vi "Autonomous Independent.vi"() -> ()   [LabVIEW 2016]
doc: "This VI is called when autonomous begins, and will automatically be terminated when autonomous ends. You can carry out timed or sensor driven robot movement independently without needing to return to the caller."
uses:
  <vilib>/Rock Robotics/Network Tables/NT Read String.vi
  Robot Global Data.vi
  <vilib>/Rock Robotics/Network Tables/NT Read Number.vi
  <vilib>/Rock Robotics/Network Tables/NT Write Number.vi
  <vilib>/Rock Robotics/Network Tables/NT Read Boolean.vi
  <vilib>/Rock Robotics/WPI/Utilities/WPI_GetSetVariantRefNum.vi
  <vilib>/Rock Robotics/WPI/ThirdParty/Sensors/ADIS16448 IMU/ADIS16448_IMU.lvlib
panel:
  out "Numeric":i32
  out "Reset":bool
  # "Be sure to right-click and choose Data Operations>>Make Current Value default if you want to save the array values with the VI"
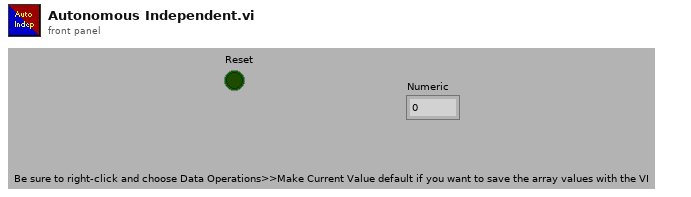
[diagram p1: front panel]
types:
  T1 = typedef "WPI_EncoderDevRef.ctl" = cluster{"DevStatus":errorcluster, "EncoderIndex":T2, "CounterIndex":T3, "DistancePerCount":dbl, "Decoding Type":T4}
  T2 = typedef "FPGA_EncoderIdx.ctl" = enum8{"Enc 0", "Enc 1", "Enc 2", "Enc 3", "Enc 4", "Enc 5", "Enc 6", "Enc 7", "Invalid"}
  T3 = typedef "FPGA_CounterCtrSystemIndex.ctl" = enum8{"Ctr 0", "Ctr 1", "Ctr 2", "Ctr 3", "Ctr 4", "Ctr 5", "Ctr 6", "Ctr 7", "Invalid"}
  T4 = typedef "WPI_EncoderType.ctl" = enum16{"1x", "2x", "4x"}
  T5 = typedef "WPI_GyroDevRef.ctl" = cluster{"DevStatus":errorcluster, "Analog Channel":T6, "Offset":dbl, "Gain (VoltsPerDegree/Second)":dbl, "Gyro Type":enum16{"Analog", "XRS450"}, "Handle":i32, "SPI Bus":T7, "Device Found":bool, "Sample Rate":dbl, "Calibrate On Open":bool}
  T6 = typedef "FPGA_AIChannel.ctl" = enum8{"AI 0", "AI 1", "AI 2", "AI 3", "AI MXP 0", "AI MXP 1", "AI MXP 2", "AI MXP 3", "Invalid"}
  T7 = typedef "spi_bus.ctl" = enum16{"SPI On-Board, CS0", "SPI On-Board, CS1", "SPI On-Board, CS2", "SPI On-Board, CS3", "SPI MXP", "Invalid"}
  T8 = typedef "ADIS16448_IMU.lvlib/ADI_IMU_ADIS16448_InterruptDevRef.ctl" = cluster{"ADI IMU DevRef":T9, "InterruptRef":T10}
  T9 = typedef "ADIS16448_IMU.lvlib/ADI_IMU_ADIS16448_IMUDevRef.ctl" = cluster{"DevStatus":errorcluster, "Handle":i32, "SPI Bus":T7, "Device Found":bool, "Device Ready":bool, "Yaw Axis":enum16{"X", "Y", "Z"}, "AHRS Algorithm":enum16{"Complementary", "Madgwick"}, "Serial":u16, "Lot ID 2":u16, "Lot ID 1":u16, "Product ID":u16}
  T10 = typedef "WPI_InterruptRef.ctl" = cluster{"DevStatus":errorcluster, "InterruptIndex":T11}
  T11 = typedef "FPGA_InterruptIndex.ctl" = enum8{"0", "1", "2", "3", "4", "5", "6", "7", "Invalid"}
  T12 = typedef "WPI_RobotDriveDevRef.ctl" = cluster{"DevStatus":errorcluster, "Motors[]":T13[], "Square Inputs":bool, "Max Output":dbl}
  T13 = typedef "WPI_MotorControlDeviceRef.ctl" = cluster{"DeviceStatus":errorcluster, "Type":T14, "PWM":cluster{"PWM Channel":T15, "DeadBand":T16}, "CAN":cluster{"Device Number":u8, "SetOutput VI Ref":variant, "GetOutput VI Ref":variant, "Enable VI Ref":variant, "Disable VI Ref":variant, "Data":variant}, "Invert":bool}
  T14 = typedef "WPI_MotorControlType.ctl" = enum16{"PWM", "CAN"}
  T15 = typedef "FPGA_DIOPWMChannel.ctl" = enum8{"PWM 0", "PWM 1", "PWM 2", "PWM 3", "PWM 4", "PWM 5", "PWM 6", "PWM 7", "PWM 8", "PWM 9", "PWM MXP 0", "PWM MXP 1", "PWM MXP 2", "PWM MXP 3", "PWM MXP 4", "PWM MXP 5", "PWM MXP 6", "PWM MXP 7", "PWM MXP 8", "PWM MXP 9", "Invalid"}
  T16 = typedef "WPI_PWMDeadband.ctl" = cluster{"Name":string, "maxPositivePwm":i32, "minPositivePwm":i32, "centerPwm":i32, "maxNegativePwm":i32, "minNegativePwm":i32, "angularRange":u16}
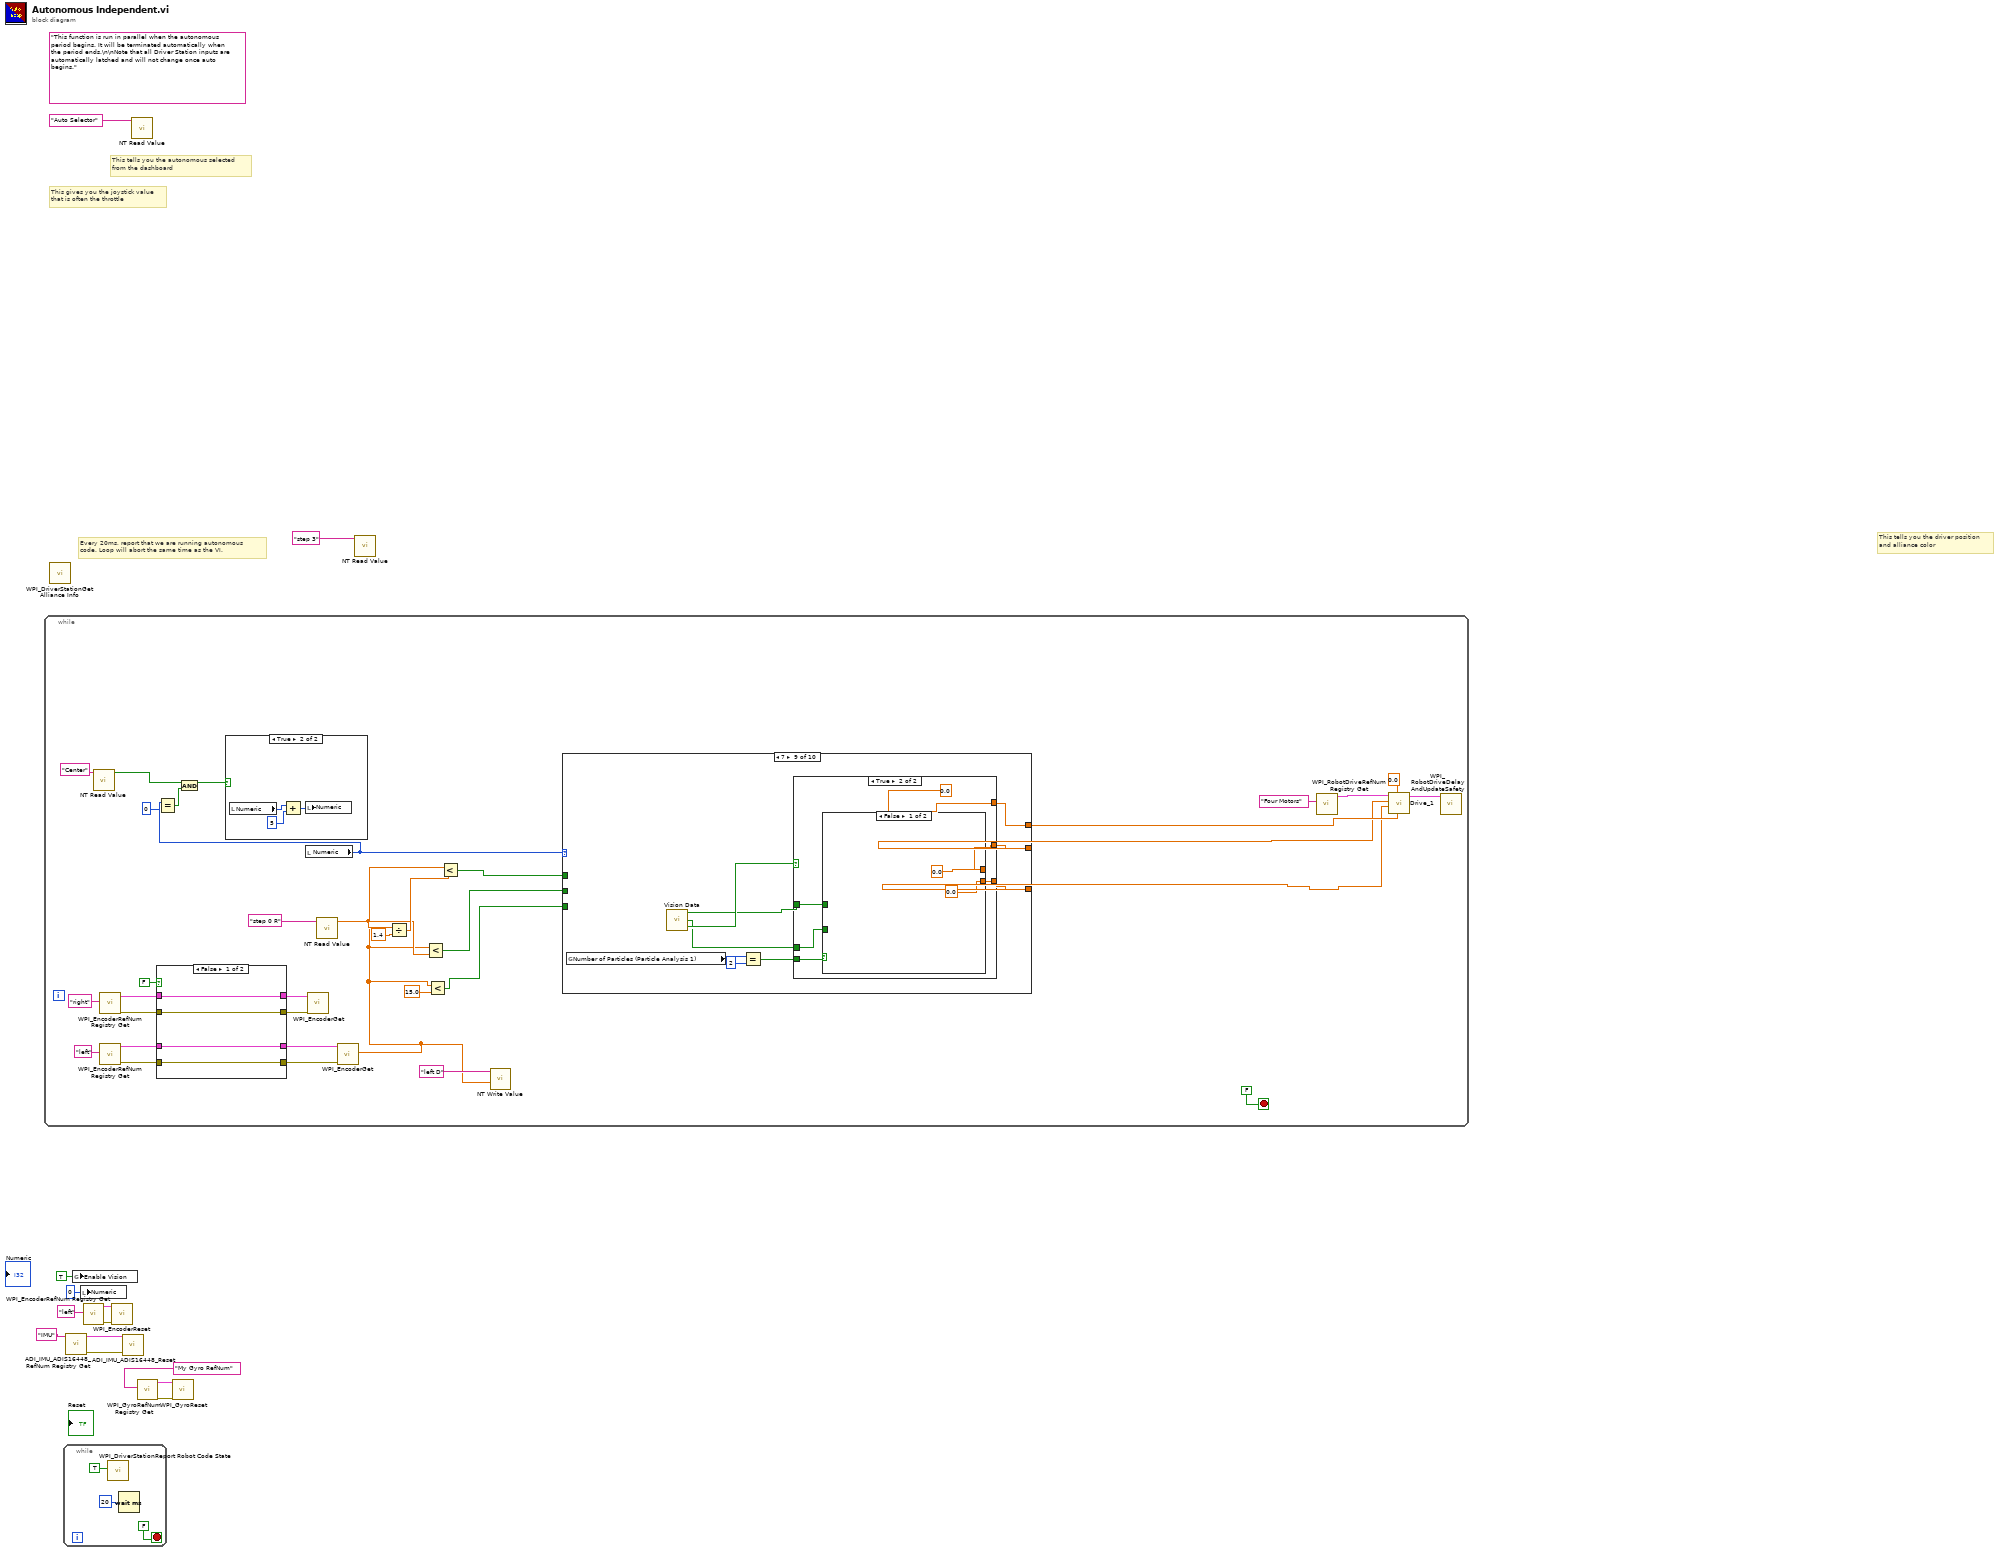
[diagram p0: block diagram]
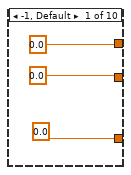
[diagram p3: hidden frame]
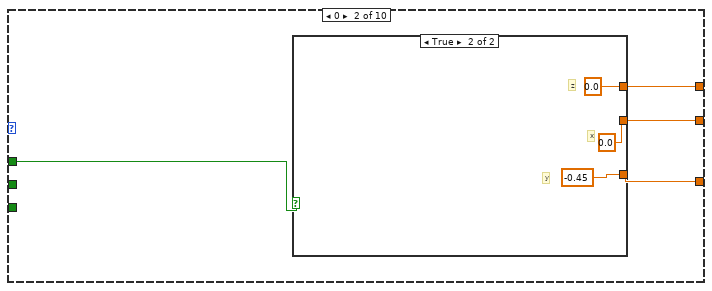
[diagram p4: hidden frame]
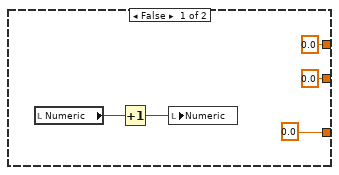
[diagram p5: hidden frame]
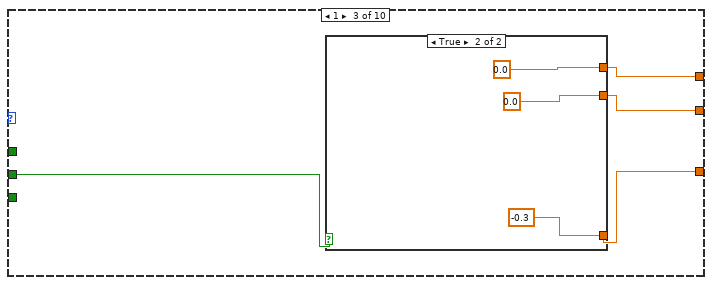
[diagram p6: hidden frame]
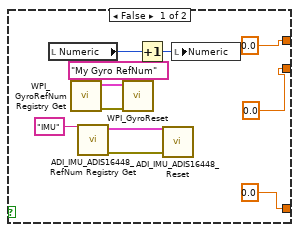
[diagram p7: hidden frame]
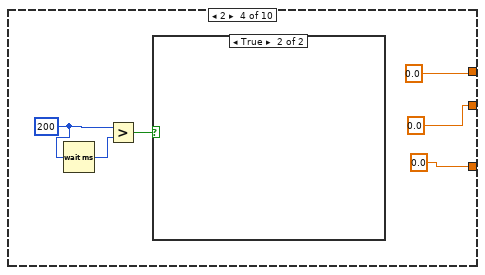
[diagram p8: hidden frame]
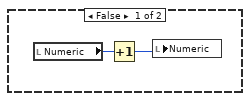
[diagram p9: hidden frame]
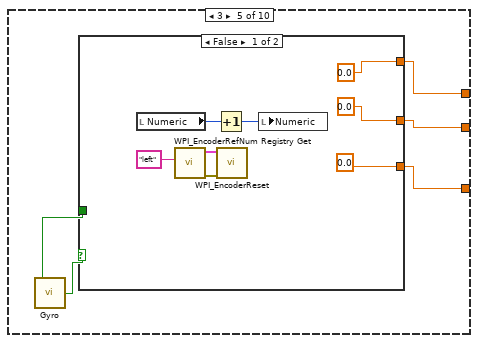
[diagram p10: hidden frame]
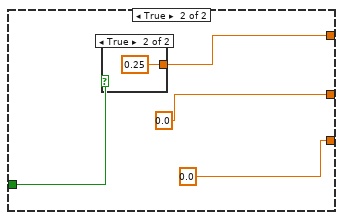
[diagram p11: hidden frame]
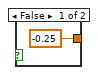
[diagram p12: hidden frame]
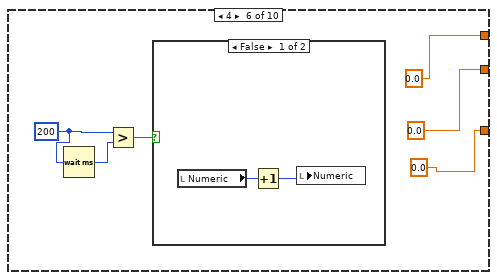
[diagram p13: hidden frame]
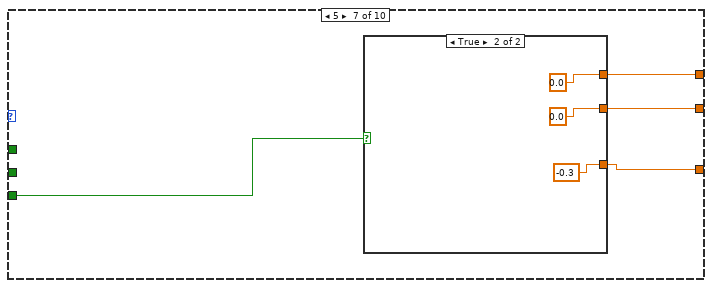
[diagram p15: hidden frame]
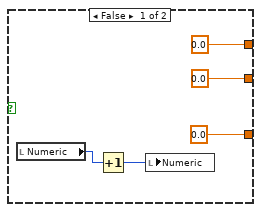
[diagram p16: hidden frame]
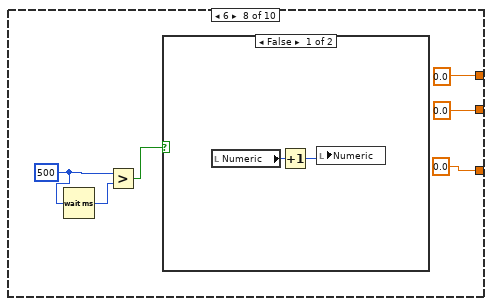
[diagram p17: hidden frame]
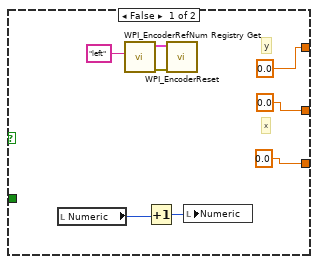
[diagram p19: hidden frame]
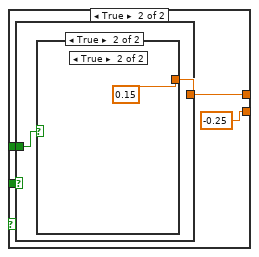
[diagram p20: hidden frame]
diagram:
  (unwired) "This function is run in parallel when the autonomous period begins. It will be terminated automatically when the period ends.\n\nNote that all Driver Station inputs are automatically latched and will not change once auto begins."
  # "This tells you the autonomous selected\nfrom the dashboard"
  # "Every 20ms, report that we are running autonomous\ncode. Loop will abort the same time as the VI."
  # "This gives you the joystick value\nthat is often the throttle"
  # "This tells you the driver position\nand alliance color"
  n1 = while {
    stop <- FALSE stop-if-true
    n2 = call-poly <vilib>:"NT Read Value.vi"("Name"="Center") -> ("Boolean"=w18:bool)  [unwired: 9 in, 1 out]
    n3 = call <vilib>:"WPI_EncoderRefNum Registry Get.vi"("refnum name"="right") -> ("error out"=w40:errorcluster, "EncoderDevRef"=w42:T1)  [unwired: 9 in]
    n4 = call <vilib>:"WPI_EncoderRefNum Registry Get.vi"("refnum name"="left") -> ("error out"=w46:errorcluster, "EncoderDevRef"=w47:T1)  [unwired: 9 in]
    n5 = case shown="False" FALSE {
      tunnel: w47 -> [w180 w188]
      tunnel: w46 -> [w179 w187]
      tunnel: [w180 w186] -> w45
      tunnel: [w179 w185] -> w44
      tunnel: [w178 w183] -> w43
      tunnel: w42 -> [w178 w184]
      tunnel: [w177 w182] -> w41
      tunnel: w40 -> [w177 w181]
      frame False {
      }
      frame True {
        n6 = call <vilib>:"WPI_EncoderReset.vi"("error in (no error)"=w181, "EncoderDevRef"=w184) -> ("error out"=w182:errorcluster, "EncoderDevRef"=w183:T1)  [unwired: 8 in]
        n7 = call <vilib>:"WPI_EncoderReset.vi"("error in (no error)"=w187, "EncoderDevRef"=w188) -> ("error out"=w185:errorcluster, "EncoderDevRef"=w186:T1)  [unwired: 8 in]
      }
    }
    n8 = local read "Numeric"() -> (w15:i32)
    n9 = Equal?(x=w15, y=0) -> (x = y?=w16:bool)
    n10 = And(x=w18, y=w16) -> (x .and. y?=w17:bool)
    n11 = case shown="True" w17 {
      frame False {
      }
      frame True {
        n12 = local read "Numeric"() -> (w51:i32)
        n13 = Add(x=w51, y=5 ("x")) -> (x+y=w49:i32)
        n14 = local write "Numeric"(w49) -> ()
      }
    }
    n15 = call <vilib>:"WPI_EncoderGet.vi"("error in (no error)"=w41, "EncoderDevRef"=w43) -> ()  [unwired: 4 in, 6 out]
    n16 = call-poly <vilib>:"NT Read Value.vi"("Name"="step 0 R") -> ("Numeric"=w32:dbl)  [unwired: 9 in, 1 out]
    n17 = call <vilib>:"WPI_EncoderGet.vi"("error in (no error)"=w44, "EncoderDevRef"=w45) -> ("Distance"=w22:dbl)  [unwired: 4 in, 5 out]
    n18 = Divide(x=w32, y=1.4) -> (x/y=w34:dbl)
    n19 = Less?(x=w22, y=w32) -> (x < y?=w24:bool)
    n20 = Less?(x=w22, y=15.0) -> (x < y?=w20:bool)
    n21 = Less?(x=w22, y=w34) -> (x < y?=w28:bool)
    n22 = call-poly <vilib>:"NT Write Value.vi"("Numeric"=w22, "Name"="left D") -> ()  [unwired: 9 in, 1 out]
    n23 = case shown="7" w15 {
      tunnel: [0.0 w58 w70 0.0 w97 0.0 w122 0.0 w146 0.0] -> w27
      tunnel: [0.0 w57 w69 0.0 w96 0.0 w121 0.0 w145 0.0] -> w26
      tunnel: [0.0 w56 w68 0.0 w95 0.0 w120 0.0 w144 -0.2] -> w25
      tunnel: w28 -> [_ w55 _ _ _ _ _ _ _ _]
      tunnel: w24 -> [_ _ w67 _ _ _ _ _ _ _]
      tunnel: w20 -> [_ _ _ _ _ _ w123 _ _ _]
      frame -1, Default {
      }
      frame 0 {
        n24 = case shown="True" w55 {
          tunnel: [0.0 0.0] -> w57
          tunnel: [0.0 0.0] -> w58
          tunnel: [0.0 -0.45] -> w56
          frame False {
            n25 = local read "Numeric"() -> (w59:i32)
            n26 = Increment(x=w59) -> (x+1=w60:i32)
            n27 = local write "Numeric"(w60) -> ()
          }
          frame True {
            # "y"
            # "x"
            # "z"
          }
        }
      }
      frame 1 {
        n28 = case shown="True" w67 {
          tunnel: [0.0 -0.3] -> w68
          tunnel: [0.0 0.0] -> w70
          tunnel: [0.0 0.0] -> w69
          frame False {
            n29 = local read "Numeric"() -> (w74:i32)
            n30 = call <vilib>:"WPI_GyroRefNum Registry Get.vi"("refnum name"="My Gyro RefNum") -> ("error out"=w76:errorcluster, "GyroDevRef"=w77:T5)  [unwired: 9 in]
            n31 = call <vilib>:"ADI_IMU_ADIS16448_RefNum Registry Get.vi"("refnum name"="IMU") -> ("error out"=w80:errorcluster, "ADI IMU Interrupt DevRef"=w79:T8)  [unwired: 9 in]
            n32 = call <vilib>:"WPI_GyroReset.vi"("error in"=w76, "GyroDevRef"=w77) -> ()  [unwired: 8 in, 2 out]
            n33 = Increment(x=w74) -> (x+1=w75:i32)
            n34 = call <vilib>:"ADI_IMU_ADIS16448_Reset.vi"("error in"=w80, "ADI IMU Interrupt DevRef"=w79) -> ()  [unwired: 8 in, 2 out]
            n35 = local write "Numeric"(w75) -> ()
          }
          frame True {
          }
        }
      }
      frame 2 {
        w86 = u32 200 ("x")
        n36 = Wait (ms)(milliseconds to wait=w86) -> (millisecond timer value=w87:u32)
        n37 = Greater?(x=w86, y=w87) -> (0:w85:bool)
        n38 = case shown="True" w85 {
          frame False {
            n39 = local read "Numeric"() -> (w92:i32)
            n40 = Increment(x=w92) -> (x+1=w91:i32)
            n41 = local write "Numeric"(w91) -> ()
          }
          frame True {
          }
        }
      }
      frame 3 {
        n42 = call "Gyro.vi"() -> ("Dis"=w93:bool, "Dir"=w94:bool)
        n43 = case shown="False" w93 {
          tunnel: [0.0 0.0] -> w95
          tunnel: [0.0 w107] -> w97
          tunnel: [0.0 0.0] -> w96
          tunnel: w94 -> [_ w108]
          frame False {
            n44 = local read "Numeric"() -> (w101:i32)
            n45 = call <vilib>:"WPI_EncoderRefNum Registry Get.vi"("refnum name"="left") -> ("error out"=w103:errorcluster, "EncoderDevRef"=w104:T1)  [unwired: 9 in]
            n46 = Increment(x=w101) -> (x+1=w102:i32)
            n47 = call <vilib>:"WPI_EncoderReset.vi"("error in (no error)"=w103, "EncoderDevRef"=w104) -> ()  [unwired: 8 in, 2 out]
            n48 = local write "Numeric"(w102) -> ()
          }
          frame True {
            n49 = case shown="True" w108 {
              tunnel: [-0.25 0.25] -> w107
              frame False {
              }
              frame True {
              }
            }
          }
        }
      }
      frame 4 {
        w116 = u32 200 ("x")
        n50 = Wait (ms)(milliseconds to wait=w116) -> (millisecond timer value=w117:u32)
        n51 = Greater?(x=w116, y=w117) -> (0:w115:bool)
        n52 = case shown="False" w115 {
          frame False {
            n53 = local read "Numeric"() -> (w119:i32)
            n54 = Increment(x=w119) -> (x+1=w118:i32)
            n55 = local write "Numeric"(w118) -> ()
          }
          frame True {
          }
        }
      }
      frame 5 {
        n56 = case shown="True" w123 {
          tunnel: [0.0 0.0] -> w122
          tunnel: [0.0 0.0] -> w121
          tunnel: [0.0 -0.3] -> w120
          frame False {
            n57 = local read "Numeric"() -> (w125:i32)
            n58 = Increment(x=w125) -> (x+1=w124:i32)
            n59 = local write "Numeric"(w124) -> ()
          }
          frame True {
          }
        }
      }
      frame 6 {
        w136 = u32 500 ("x")
        n60 = Wait (ms)(milliseconds to wait=w136) -> (millisecond timer value=w137:u32)
        n61 = Greater?(x=w136, y=w137) -> (0:w135:bool)
        n62 = case shown="False" w135 {
          frame False {
            n63 = local read "Numeric"() -> (w139:i32)
            n64 = Increment(x=w139) -> (x+1=w138:i32)
            n65 = local write "Numeric"(w138) -> ()
          }
          frame True {
          }
        }
      }
      frame 7 {
        n66 = global read "Robot Global Data.vi" "Number of Particles (Particle Analysis 1)"() -> (w143:i32)
        n67 = call "Vision Data.vi"() -> ("Dis"=w148:bool, "S?"=w141:bool, "S Dir"=w147:bool)
        n68 = Equal?(x=w143, y=2) -> (x = y?=w140:bool)
        n69 = case shown="True" w148 {
          tunnel: [0.0 0.0] -> w146
          tunnel: [0.0 w161] -> w145
          tunnel: [0.0 w157] -> w144
          tunnel: w141 -> [_ w160]
          tunnel: w147 -> [_ w159]
          tunnel: w140 -> [_ w158]
          frame False {
            # "y"
            # "x"
            n70 = local read "Numeric"() -> (w149:i32)
            n71 = call <vilib>:"WPI_EncoderRefNum Registry Get.vi"("refnum name"="left") -> ("error out"=w156:errorcluster, "EncoderDevRef"=w155:T1)  [unwired: 9 in]
            n72 = Increment(x=w149) -> (x+1=w150:i32)
            n73 = call <vilib>:"WPI_EncoderReset.vi"("error in (no error)"=w156, "EncoderDevRef"=w155) -> ()  [unwired: 8 in, 2 out]
            n74 = local write "Numeric"(w150) -> ()
          }
          frame True {
            n75 = case shown="False" w158 {
              tunnel: [0.0 w168] -> w161
              tunnel: w160 -> [_ w167]
              tunnel: w159 -> [_ w166]
              tunnel: [0.0 -0.25] -> w157
              frame False {
              }
              frame True {
                n76 = case shown="True" w167 {
                  tunnel: [0.0 w171] -> w168
                  tunnel: w166 -> [_ w170]
                  frame False {
                  }
                  frame True {
                    n77 = case shown="True" w170 {
                      tunnel: [-0.15 0.15] -> w171
                      frame False {
                      }
                      frame True {
                      }
                    }
                  }
                }
              }
            }
          }
        }
      }
      frame 8 {
      }
    }
    n78 = call <vilib>:"WPI_RobotDriveRefNum Registry Get.vi"("refnum name"="Four Motors") -> ("RobotDriveDevRef"=w30:T12)  [unwired: 9 in, 1 out]
    n79 = call "Drive_1.vi"("Rotation"=w27, "Gyro Angle"=0.0, "Y"=w25, "X"=w26, "RobotDriveDevRef 2"=w30) -> ("RobotDriveDevRef"=w29:T12)  [unwired: 4 in, 2 out]
    n80 = call <vilib>:"WPI_RobotDriveDelayAndUpdateSafety.vi"("RobotDriveDevRef"=w29) -> ()  [unwired: 9 in, 2 out]
  }
  n81 = call <vilib>:"WPI_DriverStationGet Alliance Info.vi"() -> ()  [unwired: 12 out]
  n82 = while {
    stop <- FALSE stop-if-true
    n83 = call <vilib>:"WPI_DriverStationReport Robot Code State.vi"("Autonomous"=TRUE) -> ()  [unwired: 10 in, 1 out]
    n84 = Wait (ms)(milliseconds to wait=u32 20) -> ()  [unwired: 1 out]
  }
  n85 = call <vilib>:"ADI_IMU_ADIS16448_RefNum Registry Get.vi"("refnum name"="IMU") -> ("error out"=w7:errorcluster, "ADI IMU Interrupt DevRef"=w8:T8)  [unwired: 9 in]
  n86 = global write "Robot Global Data.vi" "Enable Vision"(TRUE ("Enable Vision")) -> ()
  n87 = local write "Numeric"(0 ("Numeric")) -> ()
  n88 = call <vilib>:"WPI_EncoderRefNum Registry Get.vi"("refnum name"="left") -> ("error out"=w11:errorcluster, "EncoderDevRef"=w10:T1)  [unwired: 9 in]
  n89 = call <vilib>:"WPI_EncoderReset.vi"("error in (no error)"=w11, "EncoderDevRef"=w10) -> ()  [unwired: 8 in, 2 out]
  n90 = call <vilib>:"ADI_IMU_ADIS16448_Reset.vi"("error in"=w7, "ADI IMU Interrupt DevRef"=w8) -> ()  [unwired: 8 in, 2 out]
  n91 = call-poly <vilib>:"NT Read Value.vi"("Name"="Auto Selector") -> ()  [unwired: 9 in, 2 out]
  n92 = call <vilib>:"WPI_GyroRefNum Registry Get.vi"("refnum name"="My Gyro RefNum") -> ("error out"=w5:errorcluster, "GyroDevRef"=w4:T5)  [unwired: 9 in]
  n93 = call <vilib>:"WPI_GyroReset.vi"("error in"=w5, "GyroDevRef"=w4) -> ()  [unwired: 8 in, 2 out]
  n94 = call-poly <vilib>:"NT Read Value.vi"("Name"="step 3") -> ()  [unwired: 9 in, 2 out]
